vi "TimeInterpRotation_New.vi"(11 "MaxTime":dbl=1.0) -> (3 "TimeInterpRotation":T1 {"RotationValues"."SIN" format="%13.4f"; "RotationValues"."COS" format="%13.4f"; "RotationValues"."VALUE" format="%13.4f"})   [LabVIEW 2019, in "Trajectory_Library.lvlib"]
doc: "Inputs:\n - \n\nOutputs:\n - Function Generator -- Created data structure"
uses:
  Trajectory_Library.lvlib
  ROTATION2D.ctl
  TIME_INTERPOLATABLE_ROTATION.ctl
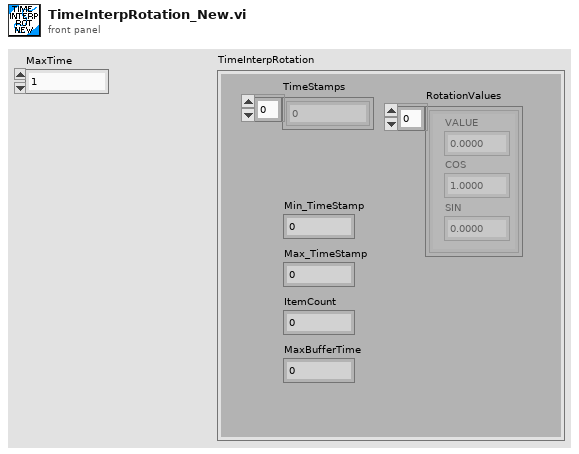
[diagram p1: front panel]
types:
  T1 = typedef "Trajectory_Library.lvlib/TIME_INTERPOLATABLE_ROTATION.ctl" = cluster{"TimeStamps":dbl[], "RotationValues":T2[], "Min_TimeStamp":dbl, "Max_TimeStamp":dbl, "ItemCount":i32, "MaxBufferTime":dbl}
  T2 = typedef "Trajectory_Library.lvlib/ROTATION2D.ctl" = cluster{"VALUE":dbl, "COS":dbl, "SIN":dbl}
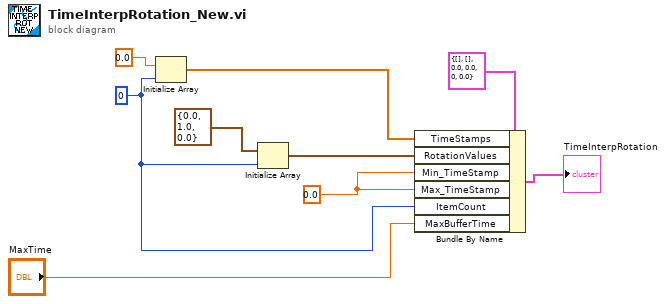
[diagram p0: block diagram]
diagram:
  w6 = 0.0 ("X")
  w2 = 0 ("dimension size")
  n1 = Initialize Array(0.0 ("element"), w2) -> (w7:dbl[])
  n2 = Initialize Array(T2 {"VALUE"=0.0, "COS"=1.0, "SIN"=0.0} ("ROTATION"), w2) -> (w3:T2[])
  n3 = Bundle By Name(cluster=T1 {"TimeStamps"=[], "RotationValues"=[], "Min_TimeStamp"=0.0, "Max_TimeStamp"=0.0, "ItemCount"=0, "MaxBufferTime"=0.0} ("TIME_INTERPOLATABLE_ROTATION"), "TimeStamps"=w7, "RotationValues"=w3, "Min_TimeStamp"=w6, "Max_TimeStamp"=w6, "ItemCount"=w2, "MaxBufferTime"="MaxTime") -> (→"TimeInterpRotation":T1)
